vi "get_position.vi"(1 "INPUT":string) -> (0 "READ":string)   [LabVIEW 2016]
panel:
  out "Computer Data":dbl[](array[numeric])
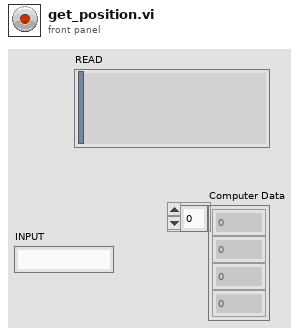
[diagram p1: front panel]
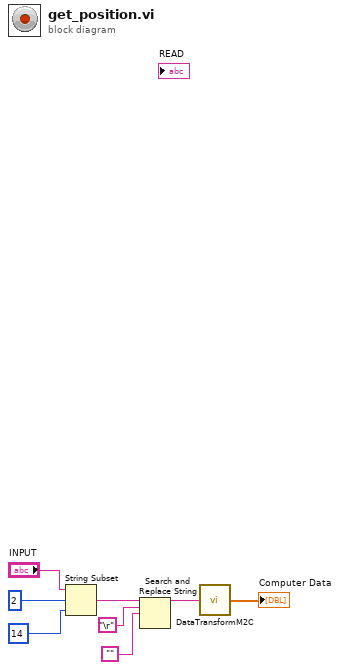
[diagram p0: block diagram]
diagram:
  n1 = String Subset(string="INPUT", offset (0)=2, length (rest)=14 ("length (rest)")) -> (substring=w4:string)
  n2 = Search and Replace String(input string=w4, search string="\r", replace string="") -> (result string=w2:string)  [unwired: 5 in, 3 out]
  n3 = call "DataTransformM2C.vi"("MotorData"=w2) -> ("Computer Data"=→"Computer Data":dbl[])
